vi "RunPowerScan.vi"(0 "object in":refnum<class "InstrumentBase.lvclass">, 5 "error in (no error)":errorcluster) -> (14 "object out":refnum<class "InstrumentBase.lvclass">, 16 "PowerScanComplete":bool, 17 "PowerScanResult":cluster{"PwrMeasured":dbl[], "PwrFreq":dbl[]}, 18 "Channels array":waveform(dbl)[](array[waveform]), 19 "error out":errorcluster)   [LabVIEW 2019, in "InstrumentBase.lvclass"]
uses:
  InstrumentBase.lvclass
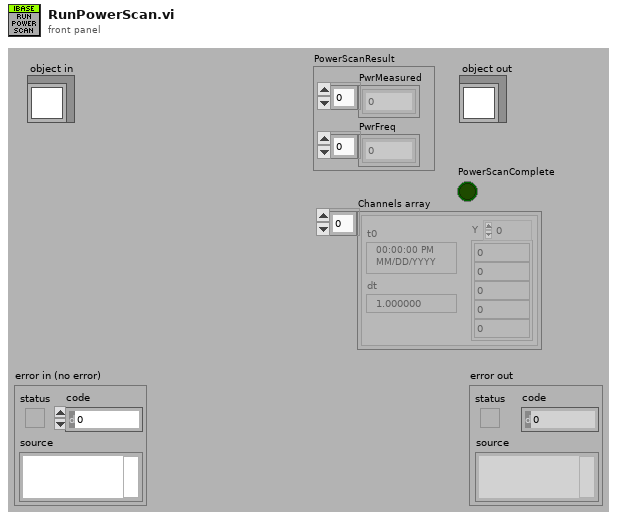
[diagram p1: front panel]
types:
  T1 = cluster{"Message":string, "Message Data":variant}
  T2 = cluster{"FreqStart(Hz)":dbl, "FreqStart(Hz)":dbl}
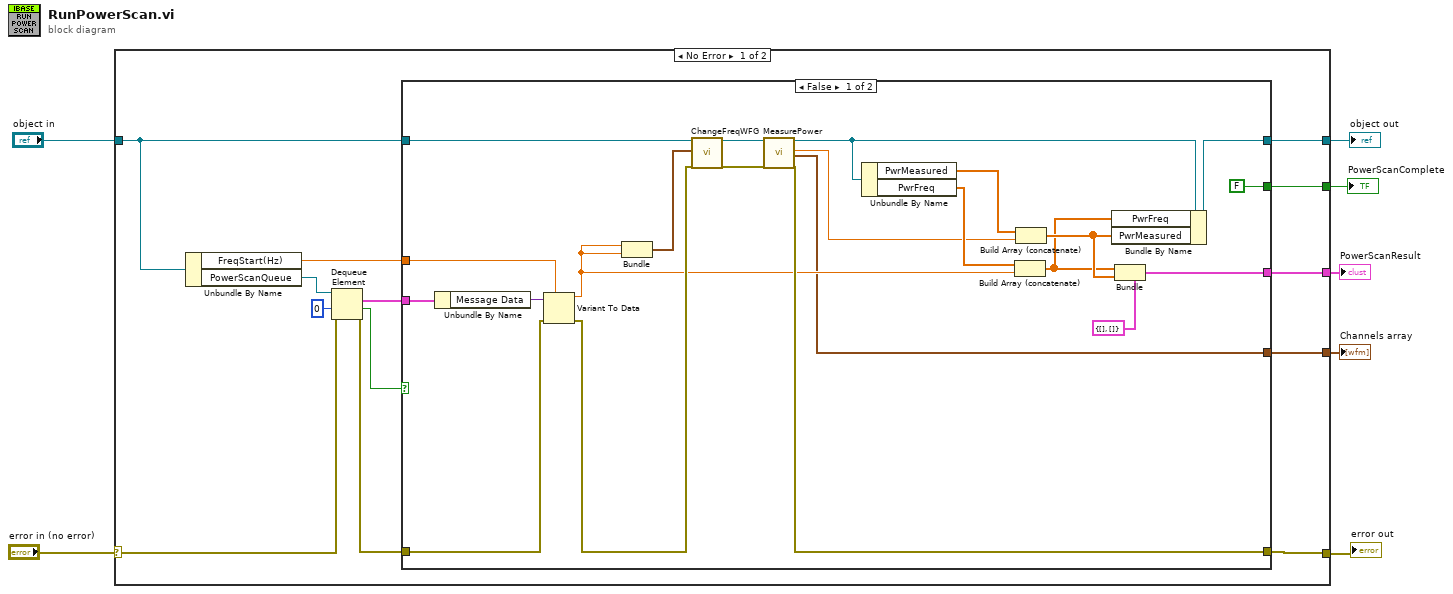
[diagram p0: block diagram]
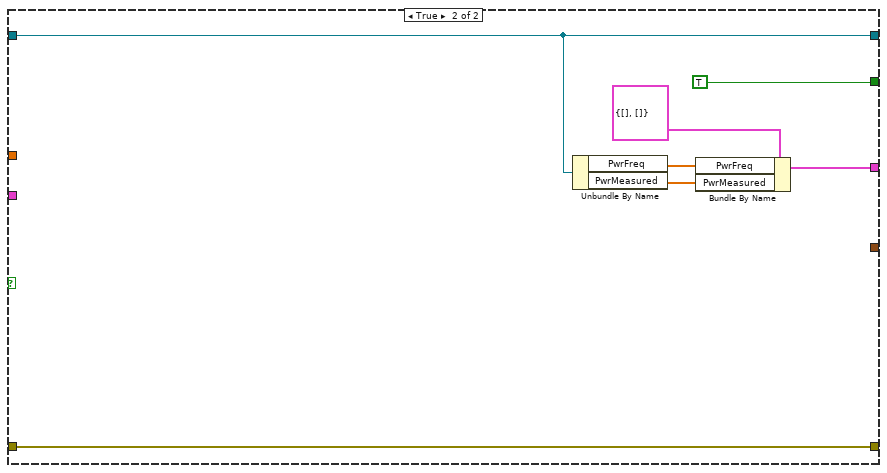
[diagram p2: hidden frame]
diagram:
  n1 = case shown="No Error" "error in (no error)" {
    selector: "error in (no error)" -> [w14 w51]
    tunnel: [w15 w51] -> w6
    tunnel: [w11 w50] -> w4
    tunnel: "object in" -> [w12 w50]
    tunnel: [w10 _] -> w3
    tunnel: [w9 _] -> w2
    tunnel: [w8 _] -> w1
    frame No Error {
      n2 = Unbundle By Name(w12) -> ("FreqStart(Hz)"=w17:dbl, "PowerScanQueue"=w20:refnum<queue>)
      n3 = Dequeue Element(queue=w20, timeout in ms (-1)=0, error in (no error)=w14) -> (element=w16:T1, timed out?=w18:bool, error out=w13:errorcluster)  [unwired: 1 out]
      n4 = case shown="False" w18 {
        tunnel: w17 -> [w42 _]
        tunnel: w16 -> [w40 _]
        tunnel: w13 -> [w39 w49]
        tunnel: [w34 w49] -> w15
        tunnel: [w28 w47] -> w11
        tunnel: w12 -> [w22 w47]
        tunnel: [FALSE TRUE] -> w10
        tunnel: [w23 w46] -> w9
        tunnel: [w21 _] -> w8
        frame False {
          n5 = Unbundle By Name(w40) -> ("Message Data"=w41:variant)
          n6 = Variant To Data(error in=w39, type=w42, Variant=w41) -> (data=w29:dbl, error out=w36:errorcluster)
          n7 = Bundle("FreqStart(Hz)"=w29, "FreqStart(Hz)"=w29) -> (w37:T2)  [unwired: 1 in]
          n8 = call-dynamic "ChangeFreqWFG.vi"("object in"=w22, "Freq Ch1&2"=w37, "error in (no error)"=w36) -> ("object out"=w26:refnum<class "InstrumentBase.lvclass">, "error out"=w35:errorcluster)  [unwired: 15 in]
          n9 = call-dynamic "MeasurePower.vi"("object in"=w26, "error in (no error)"=w35) -> ("object out"=w33:refnum<class "InstrumentBase.lvclass">, "Measured Power"=w30:dbl, "Channels array"=w21:waveform(dbl)[], "error out"=w34:errorcluster)  [unwired: 14 in]
          n10 = Unbundle By Name(w33) -> ("PwrMeasured"=w32:dbl[], "PwrFreq"=w31:dbl[])
          n11 = Build Array (concatenate)(w31, w29) -> (w25:dbl[])
          n12 = Build Array (concatenate)(w32, w30) -> (w27:dbl[])
          n13 = Bundle By Name(cluster=w33, "PwrFreq"=w25, "PwrMeasured"=w27) -> (w28:refnum<class "InstrumentBase.lvclass">)
          n14 = Bundle(cluster=cluster{"PwrMeasured":dbl[], "PwrFreq":dbl[]} {"PwrMeasured"=[], "PwrFreq"=[]} ("Cluster 2"), "PwrMeasured"=w25, "PwrFreq"=w27) -> (w23:cluster{"PwrMeasured":dbl[], "PwrFreq":dbl[]})
        }
        frame True {
          n15 = Unbundle By Name(w47) -> ("PwrFreq"=w45:dbl[], "PwrMeasured"=w43:dbl[])
          n16 = Bundle By Name(cluster=cluster{"PwrFreq":dbl[], "PwrMeasured":dbl[]} {"PwrFreq"=[], "PwrMeasured"=[]} ("Cluster 2"), "PwrFreq"=w45, "PwrMeasured"=w43) -> (w46:cluster{"PwrFreq":dbl[], "PwrMeasured":dbl[]})
        }
      }
    }
    frame Error {
    }
  }
  "error out" <- w6
  "object out" <- w4
  "PowerScanComplete" <- w3
  "PowerScanResult" <- w2
  "Channels array" <- w1
